vi "AddLoadModule.vi"(0 "Config in":T1, 5 "name":string, 7 "path":string) -> (4 "Config out":T1)   [LabVIEW 2020]
uses:
  <vilib>/WebServerConfig/Config.ctl
  <vilib>/WebServerConfig/Server.ctl
  <vilib>/WebServerConfig/Alias.ctl
  <vilib>/WebServerConfig/ErrorDocument.ctl
  <vilib>/WebServerConfig/Action.ctl
  <vilib>/WebServerConfig/Redirect.ctl
  <vilib>/WebServerConfig/Interface.ctl
  <vilib>/WebServerConfig/AddHandler.ctl
  <vilib>/WebServerConfig/SSL.ctl
  <vilib>/WebServerConfig/CustomLog.ctl
  <vilib>/WebServerConfig/LoadModule.ctl
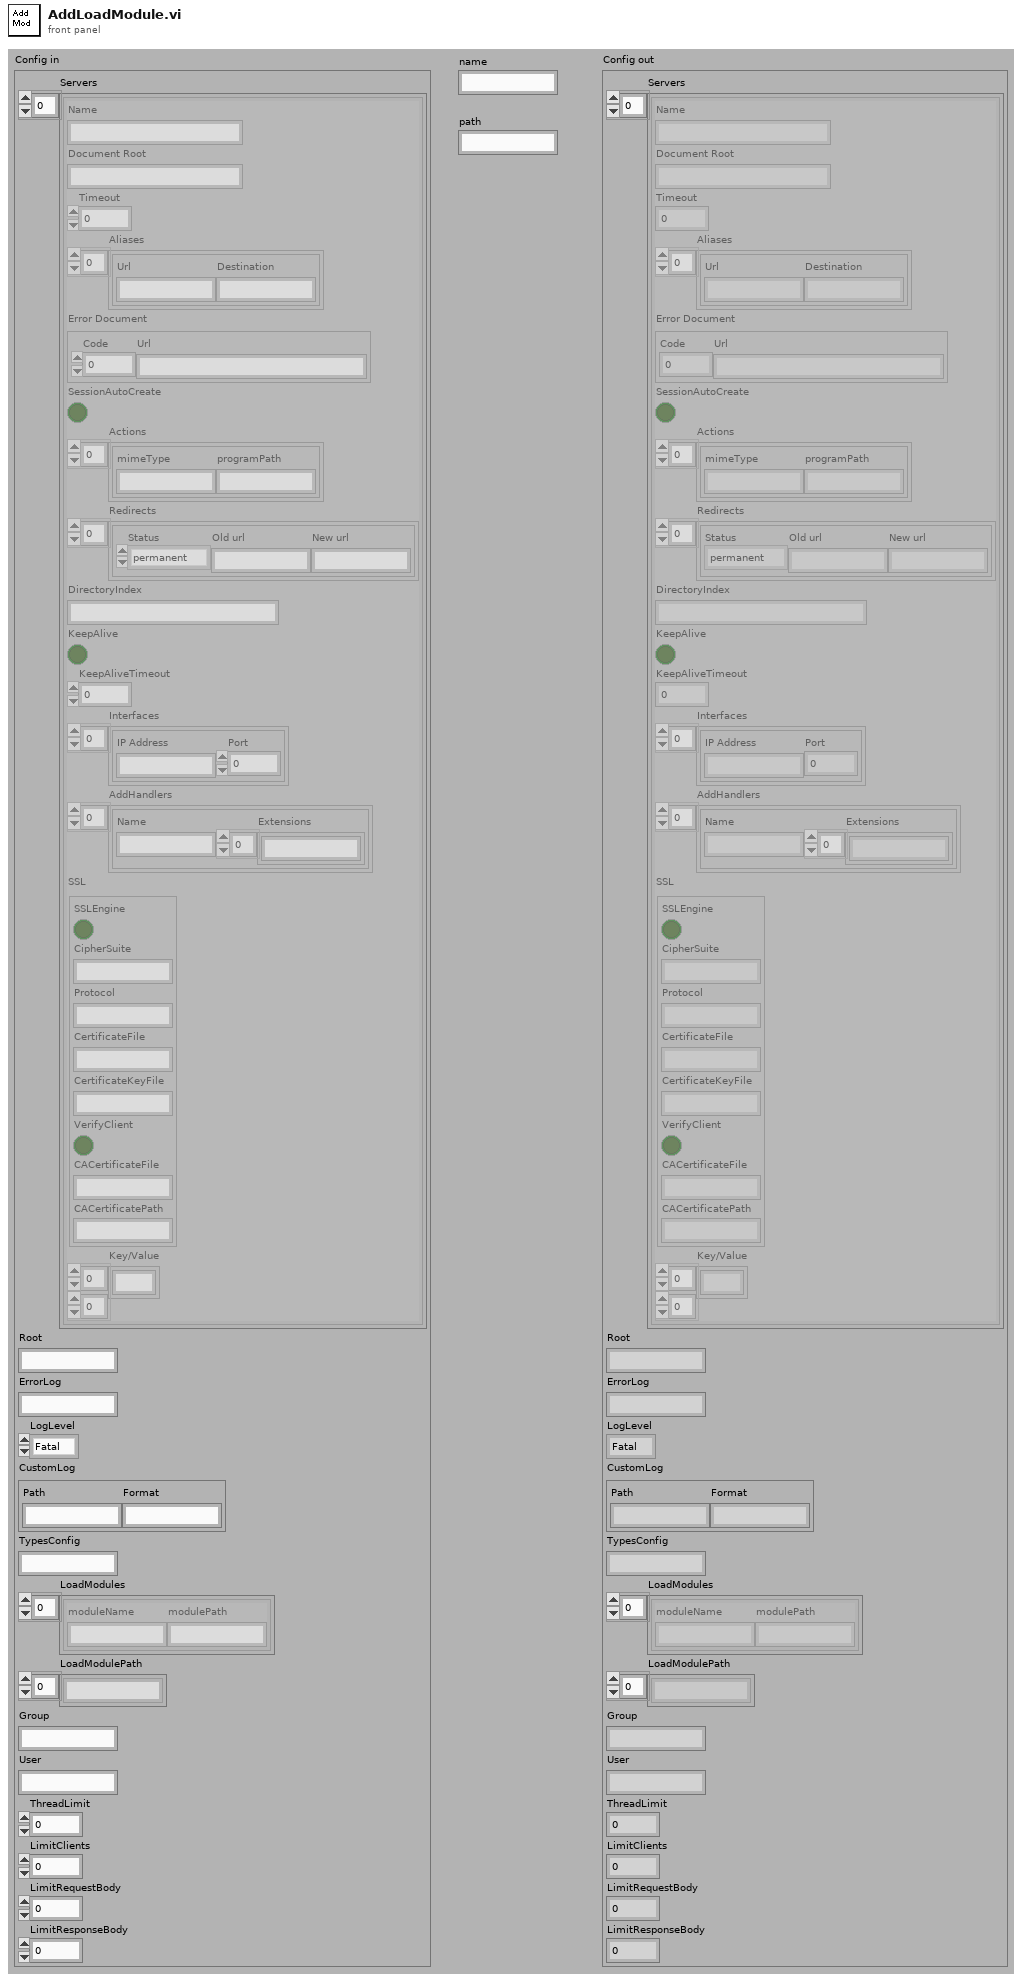
[diagram p1: front panel]
types:
  T1 = typedef "Config.ctl" = cluster{"Servers":T2[], "Root":string, "ErrorLog":string, "LogLevel":enum16{"Fatal", "Error", "Warn", "Info", "Debug", "5", "6", "7", "8", "Verbose"}, "CustomLog":T10, "TypesConfig":string, "LoadModules":T11[], "LoadModulePath":string[], "Group":string, "User":string, "ThreadLimit":u32, "LimitClients":u32, "LimitRequestBody":u32, "LimitResponseBody":u32}
  T2 = typedef "Server.ctl" = cluster{"Name":string, "Document Root":string, "Timeout":u32, "Aliases":T3[], "Error Document":T4, "SessionAutoCreate":bool, "Actions":T5[], "Redirects":T6[], "DirectoryIndex":string, "KeepAlive":bool, "KeepAliveTimeout":u32, "Interfaces":T7[], "AddHandlers":T8[], "SSL":T9, "Key/Value":string[][]}
  T3 = typedef "Alias.ctl" = cluster{"Url":string, "Destination":string}
  T4 = typedef "ErrorDocument.ctl" = cluster{"Code":u16, "Url":string}
  T5 = typedef "Action.ctl" = cluster{"mimeType":string, "programPath":string}
  T6 = typedef "Redirect.ctl" = cluster{"Status":enum16{"permanent", "temp", "seeother", "gone"}, "Old url":string, "New url":string}
  T7 = typedef "Interface.ctl" = cluster{"IP Address":string, "Port":u16}
  T8 = typedef "AddHandler.ctl" = cluster{"Name":string, "Extensions":string[]}
  T9 = typedef "SSL.ctl" = cluster{"SSLEngine":bool, "CipherSuite":string, "Protocol":string, "CertificateFile":string, "CertificateKeyFile":string, "VerifyClient":bool, "CACertificateFile":string, "CACertificatePath":string}
  T10 = typedef "CustomLog.ctl" = cluster{"Path":string, "Format":string}
  T11 = typedef "LoadModule.ctl" = cluster{"moduleName":string, "modulePath":string}
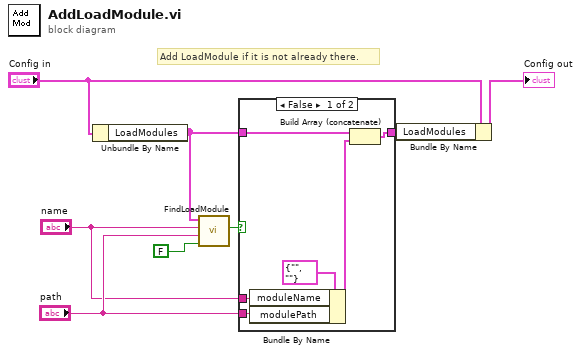
[diagram p0: block diagram]
diagram:
  # "Add LoadModule if it is not already there."
  n1 = Unbundle By Name("Config in") -> ("LoadModules"=w4:T11[])
  n2 = call <vilib>:"FindLoadModule.vi"("ByNameOnly?"=FALSE, "Path"="path", "Name"="name", "LoadModules"=w4) -> ("Found"=w6:bool)  [unwired: 7 out]
  n3 = case shown="False" w6 {
    tunnel: w4 -> [w14 w15]
    tunnel: [w13 w15] -> w3
    tunnel: "name" -> [w10 _]
    tunnel: "path" -> [w9 _]
    frame False {
      n4 = Bundle By Name(cluster=T11 {"moduleName"="", "modulePath"=""} ("LoadModule"), "moduleName"=w10, "modulePath"=w9) -> (w11:T11)
      n5 = Build Array (concatenate)(w14, w11) -> (w13:T11[])
    }
    frame True {
    }
  }
  n6 = Bundle By Name(cluster="Config in", "LoadModules"=w3) -> (→"Config out":T1)
